vi "Get Limits.vi"(7 "Axis":T1, 9 "Limits in":cluster{"Min":i64, "Max":i64}, 10 "Hailstone 2":refnum<class "Vector.lvclass">, 11 "Hailstone in":refnum<class "Vector.lvclass">) -> (2 "Limits out":cluster{"Min":i64, "Max":i64})   [LabVIEW 2021]
uses:
  Proto/Axis.ctl
  Vector.lvclass
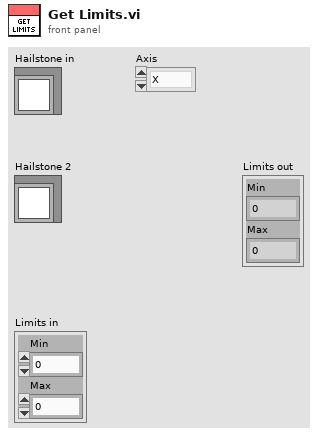
[diagram p1: front panel]
types:
  T1 = typedef "Axis.ctl" = enum16{"X", "Y", "Z"}
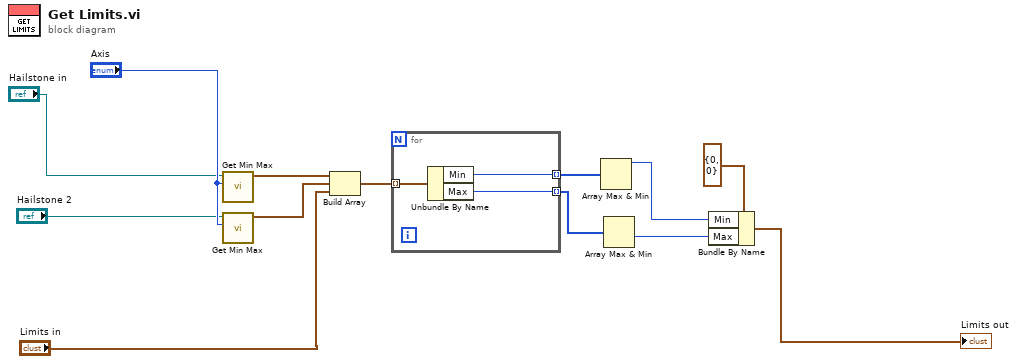
[diagram p0: block diagram]
diagram:
  n1 = call "Get Min Max.vi"("Axis"="Axis", "Hailstone in"="Hailstone in") -> ("Limits"=w2:cluster{"Min":i64, "Max":i64})  [unwired: 9 in]
  n2 = call "Get Min Max.vi"("Axis"="Axis", "Hailstone in"="Hailstone 2") -> ("Limits"=w3:cluster{"Min":i64, "Max":i64})  [unwired: 9 in]
  n3 = Build Array(w2, w3, "Limits in") -> (w4:cluster{"Min":i64, "Max":i64}[])
  n4 = for {
    tunnel: w4 -> [w16] mode=indexing
    tunnel: [w15] -> w5 mode=indexing
    tunnel: [w14] -> w6 mode=indexing
    n5 = Unbundle By Name(w16) -> ("Min"=w15:i64, "Max"=w14:i64)
  }
  n6 = Array Max & Min(array=w5) -> (max value=w8:i64)  [unwired: 3 out]
  n7 = Array Max & Min(array=w6) -> (min value=w9:i64)  [unwired: 3 out]
  n8 = Bundle By Name(cluster=cluster{"Min":i64, "Max":i64} {"Min"=0, "Max"=0} ("Limits"), "Min"=w8, "Max"=w9) -> (→"Limits out":cluster{"Min":i64, "Max":i64})
